vi "Test App App Process Added After Start Receives All Process Messages.vi"(8 "error in (no error)":errorcluster, 11 "Application Test In":refnum<class "Application Test.lvclass">) -> (0 "error out":errorcluster, 3 "Application Test Out":refnum<class "Application Test.lvclass">)   [LabVIEW 2020, in "Application Test.lvclass"]
uses:
  Application Test.lvclass
  <vilib>/Asteme/LUnit/Test Case.lvclass
  Framework/Application/Application.lvclass
  Mock Process/Mock Process.lvclass
  Framework/Process/Process.lvclass
  C:/Users/anton/Documents/GitHub/Triarc-Framework/source/Framework/Process/Process.lvclass
  C:/Users/anton/Documents/GitHub/Triarc-Framework/source/Framework/Base/Base.lvclass
  C:/Users/anton/Documents/GitHub/Triarc-Framework/source/Framework/Configuration File/Configuration File.lvclass
  C:/Users/anton/Documents/GitHub/Triarc-Framework/source/Framework/Error Handler Interface/Error Handler Interface.lvclass
  C:/Users/anton/Documents/GitHub/Triarc-Framework/source/Framework/Application/Application.lvclass
  C:/Users/anton/Documents/GitHub/Triarc-Framework/source/Framework Test/Mock Process/Mock Process.lvclass
  C:/Users/anton/Documents/GitHub/Triarc-Framework/source/Framework/Helper Loop/Helper Loop.lvclass
  C:/Users/anton/Documents/GitHub/Triarc-Framework/source/Framework Test/Process Test/Process Test.lvclass
  C:/Users/anton/Documents/GitHub/Triarc-Framework/source/Framework Test/Base Class Test/Base Test.lvclass
  C:/Program Files (x86)/National Instruments/LabVIEW 2020/vi.lib/Asteme/LUnit/Test Case.lvclass
  C:/Users/anton/Documents/GitHub/Triarc-Framework/source/Framework Test/Application Test/Application Test.lvclass
panel:
  out "Messages":string[](array[string])
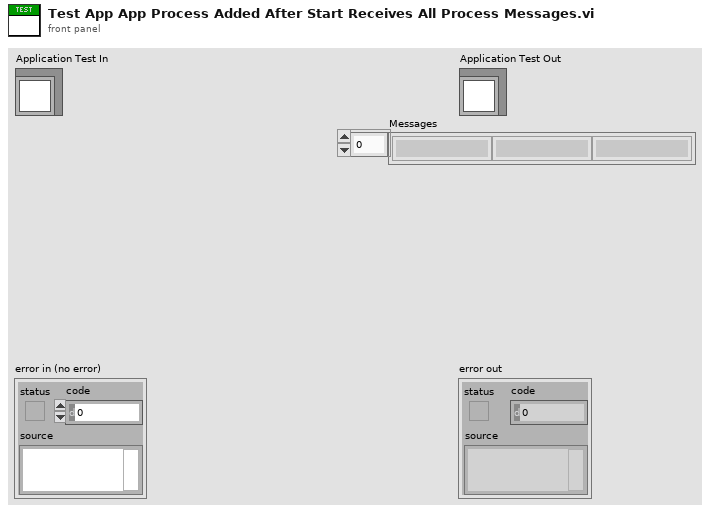
[diagram p1: front panel]
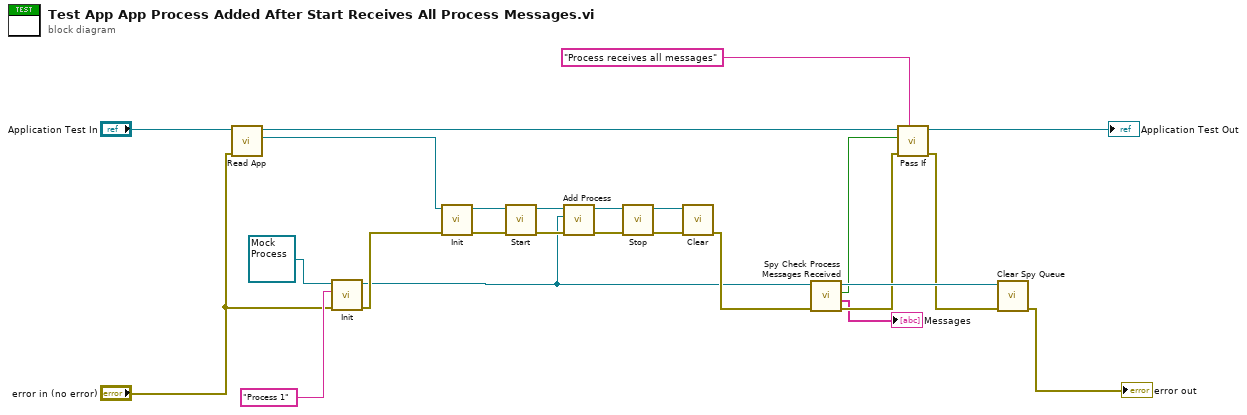
[diagram p0: block diagram]
diagram:
  n1 = call "Read App.vi"("error in (no error)"="error in (no error)", "Application Test In"="Application Test In") -> ("App out"=w16:refnum<class "Application.lvclass">, "Application Test Out"=w24:refnum<class "Application Test.lvclass">)  [unwired: 7 in, 1 out]
  n2 = call-dynamic "Init.vi"("error in (no error)"="error in (no error)", "Name"="Process 1", "Mock Process In"=refnum<class "Mock Process.lvclass"> refnum ("Mock Classes.lvlib:Mock Process.lvclass")) -> ("error out"=w19:errorcluster, "Mock Process Out"=w1:refnum<class "Mock Process.lvclass">)  [unwired: 7 in]
  n3 = call-dynamic "Init.vi"("error in (no error)"=w19, "Process In"=w16) -> ("error out"=w22:errorcluster, "Process Out"=w23:refnum<class "Application.lvclass">)  [unwired: 8 in]
  n4 = call "Start.vi"("error in (no error)"=w22, "Process In"=w23) -> ("error out"=w11:errorcluster, "Process Out"=w14:refnum<class "Application.lvclass">)  [unwired: 8 in]
  n5 = call "Add Process.vi"("error in (no error)"=w11, "Process"=w1, "Rig In"=w14) -> ("error out"=w12:errorcluster, "Rig Out"=w13:refnum<class "Application.lvclass">)  [unwired: 7 in]
  n6 = call "Stop.vi"("error in (no error)"=w12, "Process In"=w13) -> ("error out"=w20:errorcluster, "Process Out"=w21:refnum<class "Application.lvclass">)  [unwired: 7 in, 1 out]
  n7 = call-dynamic "Clear.vi"("error in (no error)"=w20, "Application In"=w21) -> ("error out"=w17:errorcluster)  [unwired: 8 in, 1 out]
  n8 = call "Spy Check Process Messages Received.vi"("error in (no error)"=w17, "Mock Process In"=w1) -> ("error out"=w8:errorcluster, "Messages"=→"Messages":string[], "Messages received?"=w6:bool, "Mock Process Out"=w10:refnum<class "Mock Process.lvclass">)  [unwired: 6 in]
  n9 = call <vilib>:"Pass If.vi"("Description"="Process receives all messages", "error in (no error)"=w8, "Pass?"=w6, "Test Case In"=w24) -> ("error out"=w7:errorcluster, "Test Case Out"=→"Application Test Out":refnum<class "Application Test.lvclass">)  [unwired: 6 in]
  n10 = call-dynamic "Clear Spy Queue.vi"("error in (no error)"=w7, "Mock Process In"=w10) -> ("error out"=→"error out":errorcluster)  [unwired: 8 in, 1 out]
